vi "Post Loop Operations.vi"(8 "error in (no error)":errorcluster, 10 "References":T1) -> (0 "error out":errorcluster)   [LabVIEW 2014, in "Initialization and IO Node Scripting.lvlib"]
uses:
  Initialization and IO Node Scripting.lvlib
  Supporting VIs/References.ctl
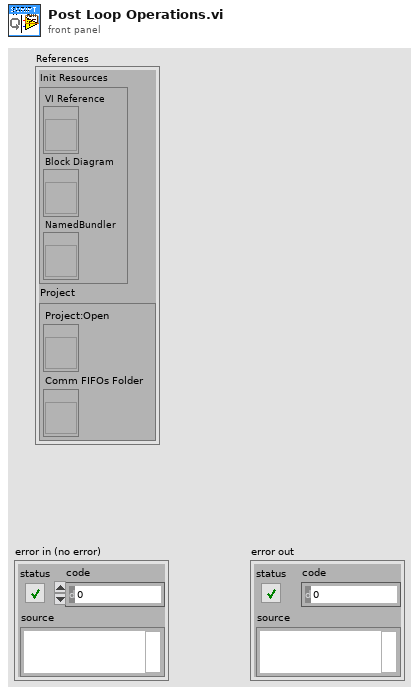
[diagram p1: front panel]
types:
  T1 = typedef "Initialization and IO Node Scripting.lvlib/References.ctl" = cluster{"Init Resources":cluster{"VI Reference":refnum<vi>, "Block Diagram":refnum<vi>, "NamedBundler":refnum<vi>}, "Project":cluster{"Project:Open":refnum<vi>, "Comm FIFOs Folder":refnum<vi>}}
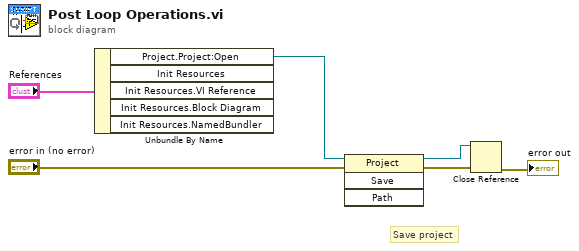
[diagram p0: block diagram]
diagram:
  # "Save project"
  n1 = Unbundle By Name("References") -> ("Project.Project:Open"=w4:refnum<vi>)  [unwired: 4 out]
  n2 = invoke class="Project" method="Save"(reference=w4, error in="error in (no error)") -> (reference out=w2:refnum<vi>, error out=w1:errorcluster)  [unwired: 2 in, 2 out]
  n3 = Close Reference(reference=w2, error in (no error)=w1) -> (error out=→"error out":errorcluster)
